vi "MGCC_FntStaMach_main.vi"() -> ()   [LabVIEW 2016]
doc: "Main function for FSM in MGCC. The inputs are flags feedback from other functions and MGLCs. The outputs are the next states and updates in sensoring datas."
panel:
  out "Data Logging":bool
  out "Data loaded":bool
  in  "b_MGCC_FntStaMach_state_estimation_enable":bool
  out "On-off":bool
  out "MGCC_StaEst_Vn":dbl[][](array[numeric])
  out "MGCC_StaEst_An":dbl[][](array[numeric])
  in  "b_MGCC_FntStaMach_All_Loop_Stop":bool
  out "Functions":bool[](array[boolean])
  out "Current state":string
  out "Current Time":string
  in  "Manual turn off":bool
  in  "Event manual panel":bool
  out "Bool of state":bool[](array[boolean])
  # "Finte State Machine"
  # "State Esimation"
  # "Model Management"
  # "Data Logging"
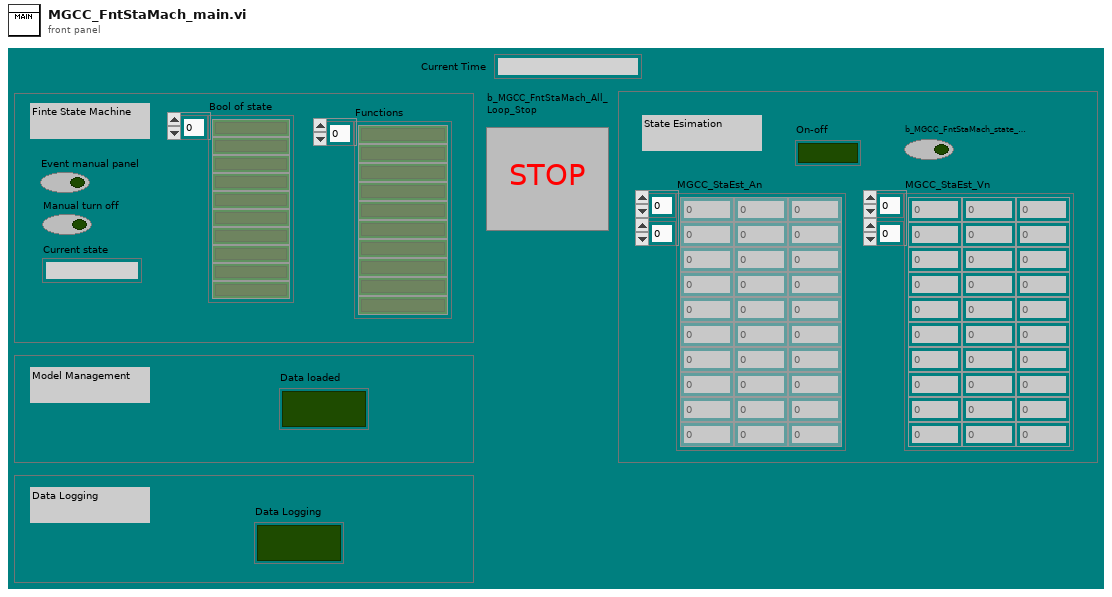
[diagram p1: front panel]
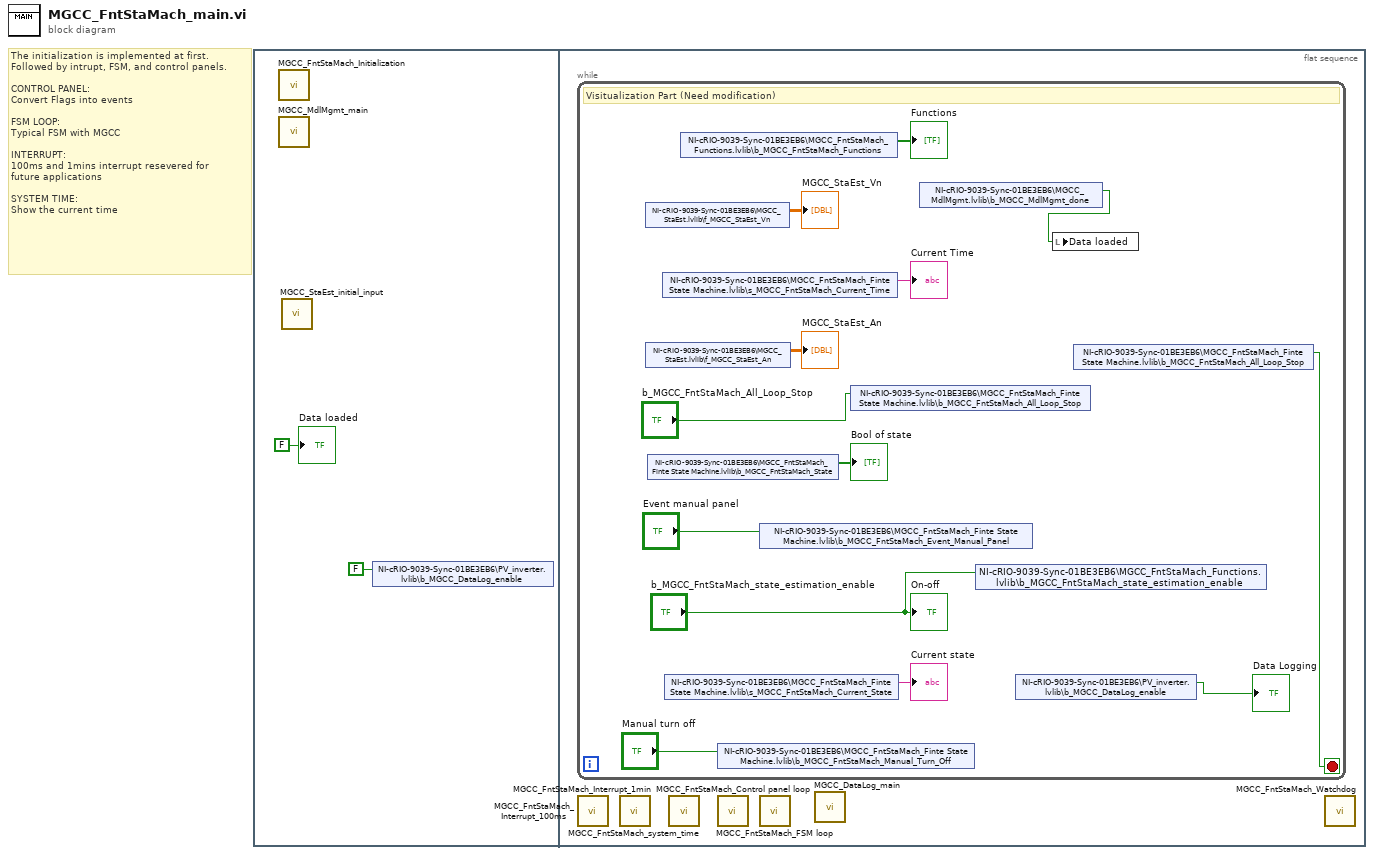
[diagram p0: block diagram]
diagram:
  # "The initialization is implemented at first.\nFollowed by intrupt, FSM, and control panels.\n\nCONTROL PANEL:\nConvert Flags into events\n\nFSM LOOP:\nTypical FSM with MGCC\n\nINTERRUPT:\n100ms and 1mins interrupt resevered for \nfuture applications\n\nSYSTEM TIME:\nShow the current time"
  n1 = flat-sequence {
    frame #0 {
      n2 = call "MGCC_FntStaMach_Initialization.vi"() -> ()  [unwired: 12 in]
      n3 = call "MGCC_MdlMgmt_main.vi"() -> ()  [unwired: 12 in]
      n4 = call "MGCC_StaEst_initial_input.vi"() -> ()  [unwired: 12 in]
      n5 = shared-variable "NI-cRIO-9039-Sync-01BE3EB6\\PV_inverter.lvlib\\b_MGCC_DataLog_enable"(FALSE ("b_MGCC_DataLog_enable")) -> ()  [unwired: 1 in, 1 out]
      "Data loaded" <- FALSE ("Data loaded")
    }
    frame #1 {
      n6 = while {
        stop <- w14 stop-if-true
        # "Visitualization Part (Need modification)"
        n7 = shared-variable "NI-cRIO-9039-Sync-01BE3EB6\\MGCC_StaEst.lvlib\\f_MGCC_StaEst_Vn"() -> (→"MGCC_StaEst_Vn":dbl[][])  [unwired: 1 in, 1 out]
        n8 = shared-variable "NI-cRIO-9039-Sync-01BE3EB6\\MGCC_StaEst.lvlib\\f_MGCC_StaEst_An"() -> (→"MGCC_StaEst_An":dbl[][])  [unwired: 1 in, 1 out]
        n9 = shared-variable "NI-cRIO-9039-Sync-01BE3EB6\\MGCC_FntStaMach_Finte State Machine.lvlib\\b_MGCC_FntStaMach_State"() -> (→"Bool of state":bool[])  [unwired: 1 in, 1 out]
        n10 = shared-variable "NI-cRIO-9039-Sync-01BE3EB6\\MGCC_FntStaMach_Finte State Machine.lvlib\\s_MGCC_FntStaMach_Current_Time"() -> (→"Current Time":string)  [unwired: 1 in, 1 out]
        n11 = shared-variable "NI-cRIO-9039-Sync-01BE3EB6\\MGCC_FntStaMach_Finte State Machine.lvlib\\s_MGCC_FntStaMach_Current_State"() -> (→"Current state":string)  [unwired: 1 in, 1 out]
        n12 = shared-variable "NI-cRIO-9039-Sync-01BE3EB6\\MGCC_FntStaMach_Functions.lvlib\\b_MGCC_FntStaMach_Functions"() -> (→"Functions":bool[])  [unwired: 1 in, 1 out]
        n13 = shared-variable "NI-cRIO-9039-Sync-01BE3EB6\\MGCC_FntStaMach_Finte State Machine.lvlib\\b_MGCC_FntStaMach_Manual_Turn_Off"("Manual turn off") -> ()  [unwired: 1 in, 1 out]
        n14 = shared-variable "NI-cRIO-9039-Sync-01BE3EB6\\MGCC_FntStaMach_Finte State Machine.lvlib\\b_MGCC_FntStaMach_Event_Manual_Panel"("Event manual panel") -> ()  [unwired: 1 in, 1 out]
        n15 = shared-variable "NI-cRIO-9039-Sync-01BE3EB6\\MGCC_FntStaMach_Finte State Machine.lvlib\\b_MGCC_FntStaMach_All_Loop_Stop"("b_MGCC_FntStaMach_All_Loop_Stop") -> ()  [unwired: 1 in, 1 out]
        n16 = shared-variable "NI-cRIO-9039-Sync-01BE3EB6\\MGCC_MdlMgmt.lvlib\\b_MGCC_MdlMgmt_done"() -> (w4:bool)  [unwired: 1 in, 1 out]
        n17 = shared-variable "NI-cRIO-9039-Sync-01BE3EB6\\MGCC_FntStaMach_Functions.lvlib\\b_MGCC_FntStaMach_state_estimation_enable"("b_MGCC_FntStaMach_state_estimation_enable") -> ()  [unwired: 1 in, 1 out]
        n18 = shared-variable "NI-cRIO-9039-Sync-01BE3EB6\\PV_inverter.lvlib\\b_MGCC_DataLog_enable"() -> (→"Data Logging":bool)  [unwired: 1 in, 1 out]
        n19 = local write "Data loaded"(w4) -> ()
        n20 = shared-variable "NI-cRIO-9039-Sync-01BE3EB6\\MGCC_FntStaMach_Finte State Machine.lvlib\\b_MGCC_FntStaMach_All_Loop_Stop"() -> (w14:bool)  [unwired: 1 in, 1 out]
        "On-off" <- "b_MGCC_FntStaMach_state_estimation_enable"
      }
      n21 = call "MGCC_FntStaMach_Interrupt_100ms.vi"() -> ()  [unwired: 11 in, 1 out]
      n22 = call "MGCC_FntStaMach_Interrupt_1min.vi"() -> ()  [unwired: 11 in, 1 out]
      n23 = call "MGCC_FntStaMach_system_time.vi"() -> ()  [unwired: 12 in]
      n24 = call "MGCC_FntStaMach_Control panel loop.vi"() -> ()  [unwired: 12 in]
      n25 = call "MGCC_FntStaMach_FSM loop.vi"() -> ()  [unwired: 8 in, 4 out]
      n26 = call "MGCC_DataLog_main.vi"() -> ()  [unwired: 12 in]
      n27 = call "MGCC_FntStaMach_Watchdog.vi"() -> ()  [unwired: 12 in]
    }
  }
